vi "Image Analysis.vi"() -> ()   [LabVIEW 2010]
uses:
  <vilib>/Utility/miscctls.llb/LVMouseTypeDef.ctl
  <vilib>/Analysis/2dsp.llb/2D Real FFT.vi
  <vilib>/Analysis/2dsp.llb/2D Inverse Real FFT.vi
  <vilib>/picture/picture.llb/Draw True-Color Pixmap.vi
  <vilib>/Analysis/NI_AALPro.lvlib
  <vilib>/Analysis/NI_AALBase.lvlib
panel:
  in  "System Refresh Button":bool
  in  "Clear Image":bool
  in  "Find Atoms":bool
  in  "Save Marked Image":bool
  in  "index":i32
  in  "Pixel intensity":u8[][](array[numeric])
  out "Numeric 2":i32
  out "Numeric":i32
  in  "Tab Control 2":enum32{"Page 1", "Page 2"}(tab)
  in  "Local Max":bool
  in  "Pixel Radius":i32
  in  "Cutoff":dbl(slide)=0.9219858156028369 scale=0.0..1.0
  in  "STEM Image":path
  out "History Data":T1(array[cluster])
  in  "Tab Control":enum32{"Image", "FFT", "Analysis", "Advanced"}(tab)
  out "Working Image":picture
  in  "Zoom":dbl(slide)=0.9832134292565947 scale=0.0..20.0
  in  "Color":u32(colorbox)=16726826
  out "Angle (Degrees)":dbl
  out "Cos (Theta)":dbl
  in  "System Stop Button":bool
  out "Cropped Image":picture
  out "FFT":picture
  in  "Zoom 2":dbl(slide)=1.079136690647482 caption="Zoom" scale=0.0..10.0
  in  "Noise Factor":dbl(slide) scale=0.0..2.0
  in  "Xlength":i32(slide)=1024 scale=0.0..1024.0
  in  "YLength":i32(slide)=1024
  in  "X":i32
  in  "Y":i32
  in  "Mod":i32
  in  "Max X":dbl(slide) scale=0.0..1024.0
  in  "MAx Y":dbl
  out "RSD (%)":dbl format="%#_g%%"
  out "Std Dev":dbl
  out "Average Angle (Deg)":dbl
  out "Histogram Graph":T2(graph)
  out "Histogram Graph 2":T2(graph)
  out "Angles":T3(graph)
  in  "intervals":i32(slide)=10 scale=0.0..10.0
  out "RSD (%) 2":dbl format="%#_g%%"
  out "Std Dev 2":dbl
  out "Average Angle (Deg) 2":dbl
  in  "Slice Index":i32=24
  out "Atom Positions":T4(array[cluster])
  out "Last Last Mouse Pos":cluster{"Mouse X":i32, "Mouse Y":i32}
  out "Last Mouse Position":cluster{"Mouse X":i32, "Mouse Y":i32}={"Mouse X"=-1, "Mouse Y"=-1}
  out "CdTe Position Vector":dbl[](array[numeric])
  out "Mouse":T5={"Mouse Position"={"X"=21, "Y"=535}, "Mouse Modifiers"={"Button Down"=FALSE, "Shift Mod"=FALSE, "Menu Mod"=FALSE, "Option Mod"=FALSE}}
  out "Original Image":picture
  # "Drag and drop an Image here"
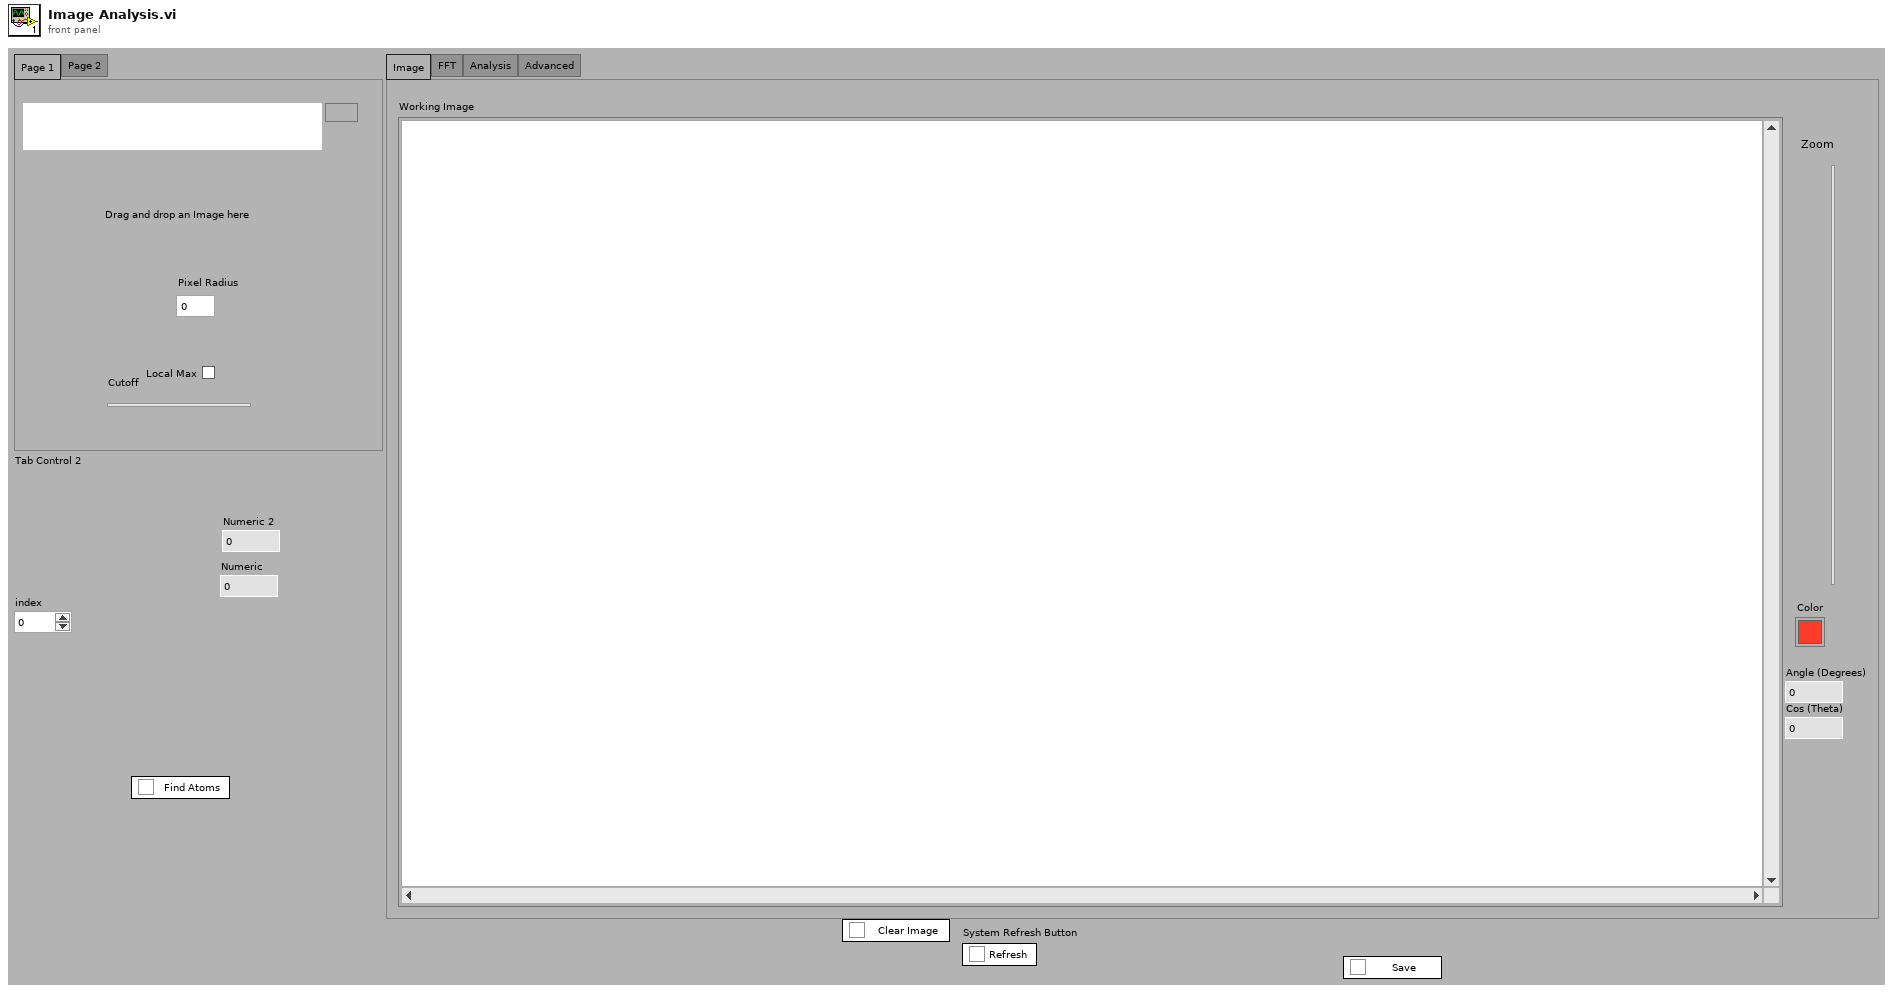
[diagram p1: front panel]
types:
  T1 = cluster{"Angle (Degrees)":dbl, "Cos (Theta)":dbl}[]
  T2 = cluster{"X Values":dbl[], "Histogram: h(x)":i32[]}
  T3 = cluster{"Angle (Degrees)":dbl, "Cos (Theta)":dbl}
  T4 = cluster{"Atom":string, "Pixel X":i32, "Pixel Y":i32}[]
  T5 = typedef "LVMouseTypeDef.ctl" = cluster{"Mouse Position":cluster{"X":i32, "Y":i32}, "Mouse Modifiers":cluster{"Button Down":bool, "Shift Mod":bool, "Menu Mod":bool, "Option Mod":bool}}
  T6 = cluster{"Width":u16, "Style":enum32{"Solid", "Dash", "Dot", "DashDot", "DashDotDot"}}
  T7 = typedef "imagedata.ctl" = cluster{"image type":i32, "image depth":i32, "image":u8[], "mask":u8[], "colors":u32[], "Rectangle":cluster{"left":i16, "top":i16, "right":i16, "bottom":i16}}
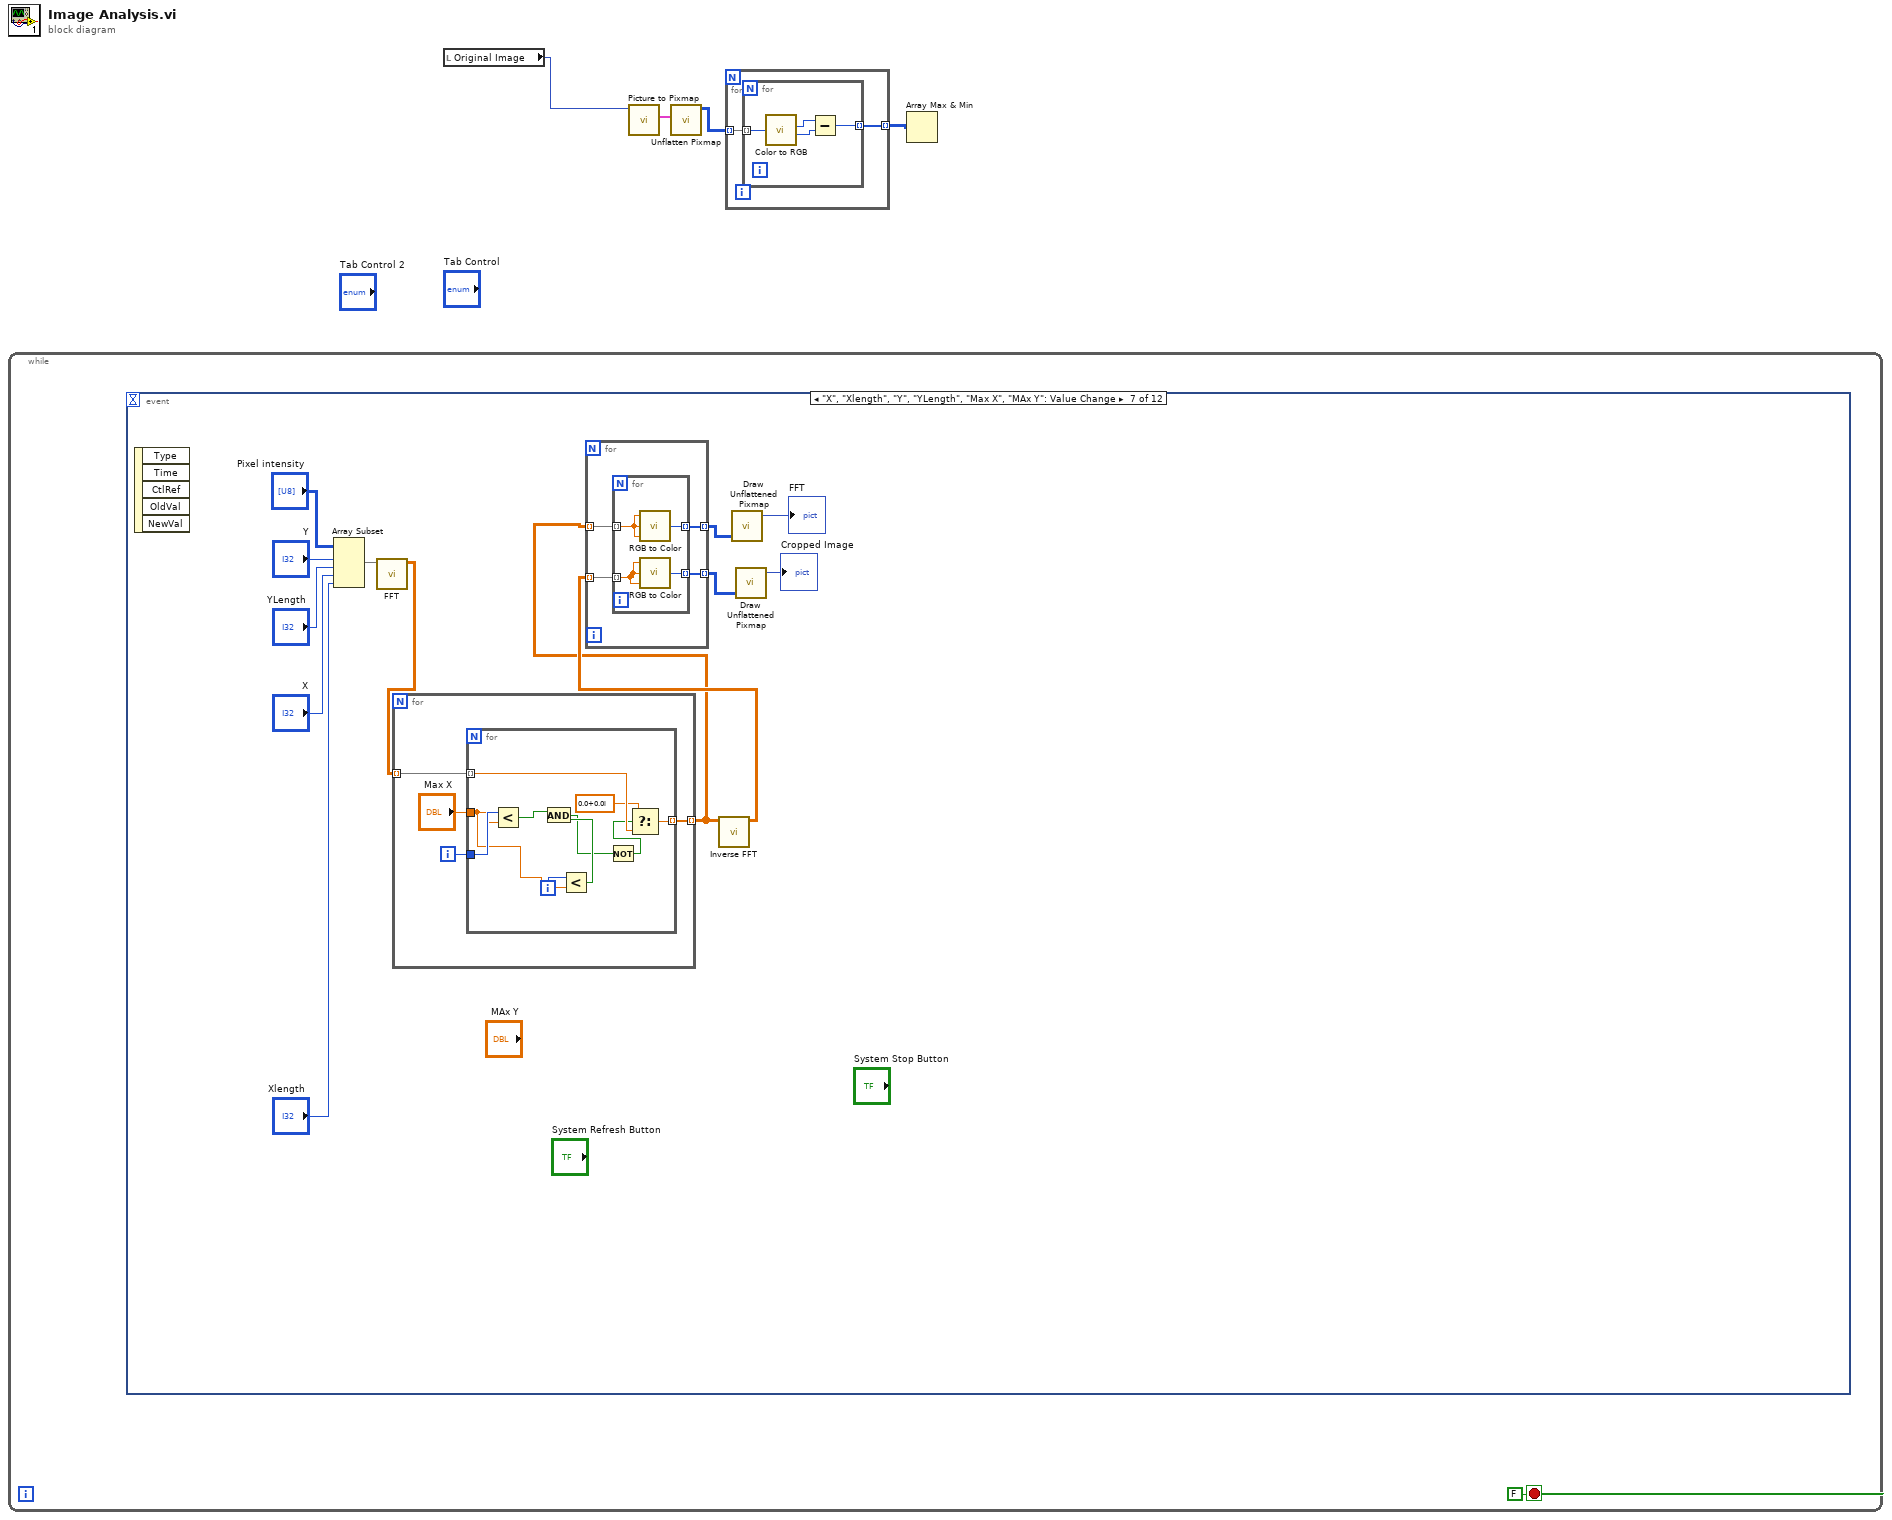
[diagram p0: block diagram]
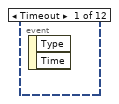
[diagram p2: hidden frame]
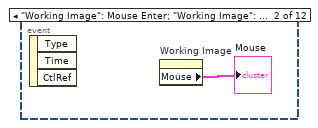
[diagram p3: hidden frame]
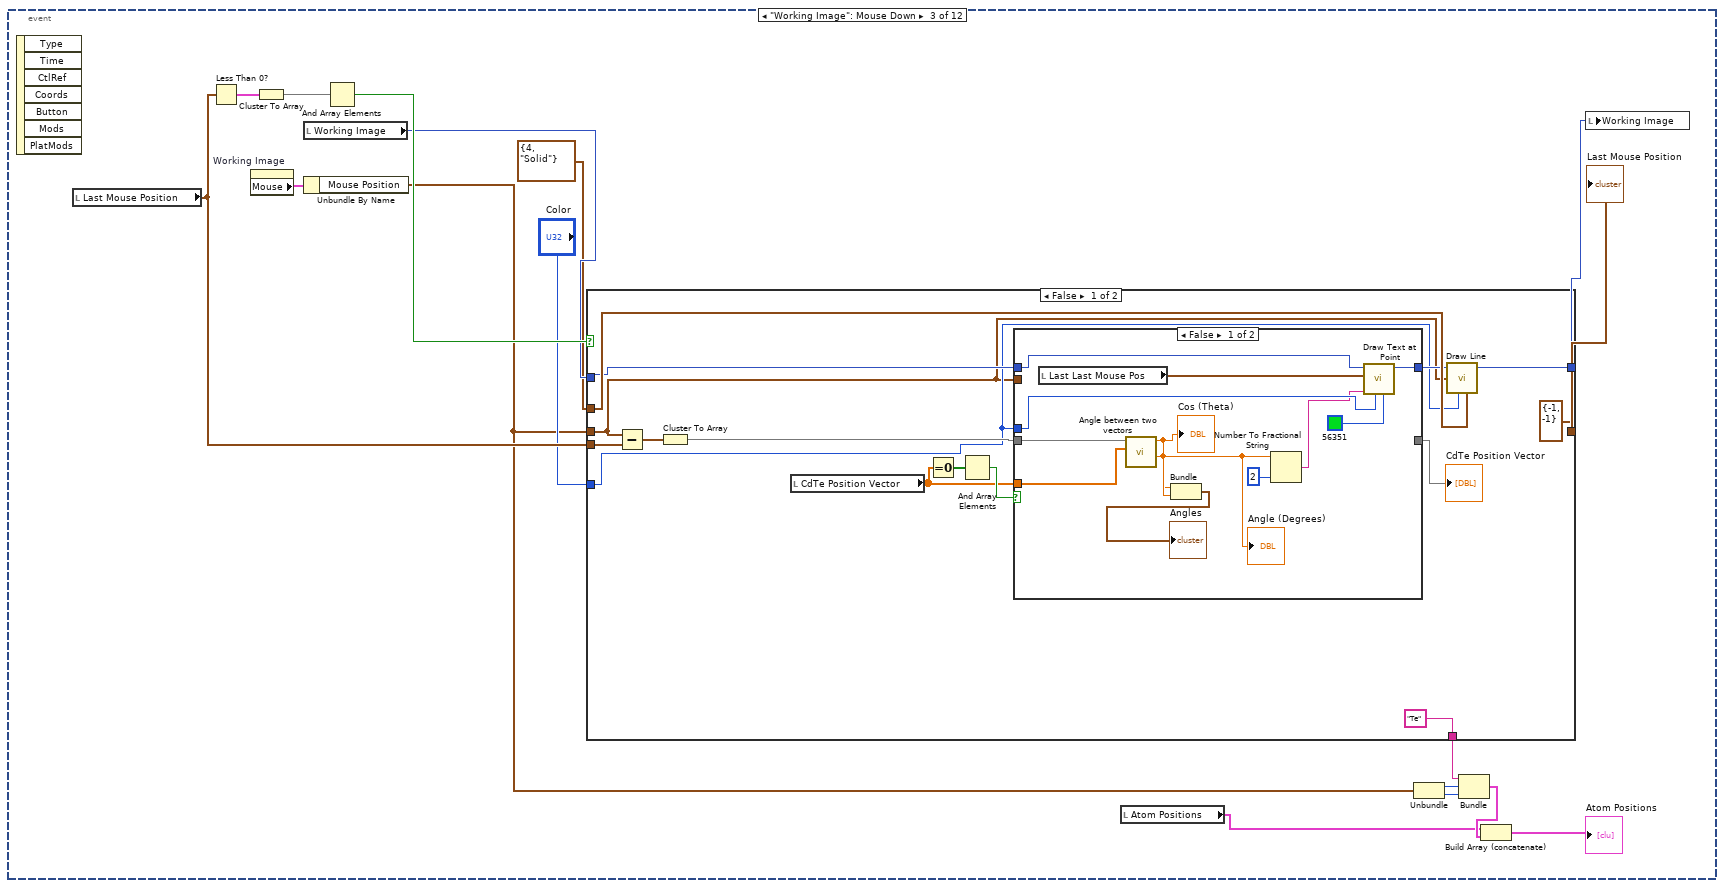
[diagram p4: hidden frame]
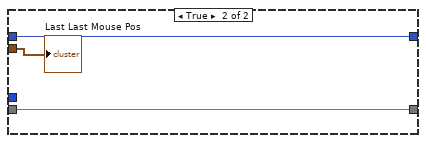
[diagram p5: hidden frame]
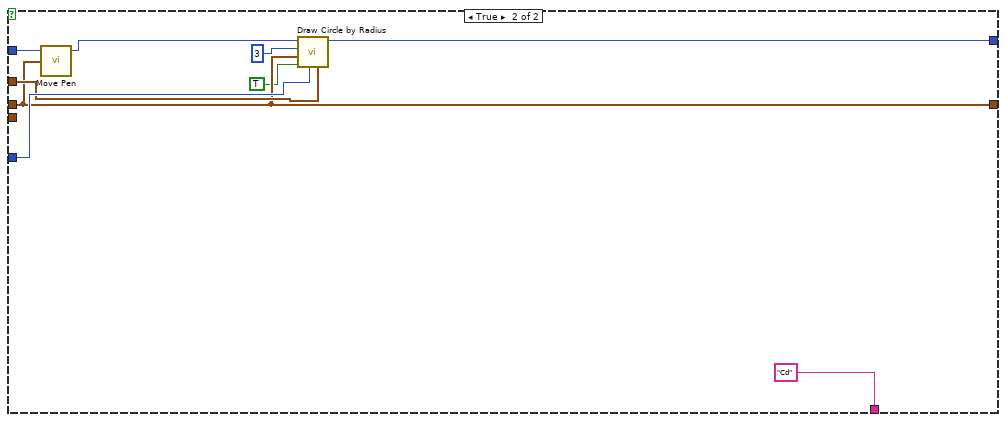
[diagram p6: hidden frame]
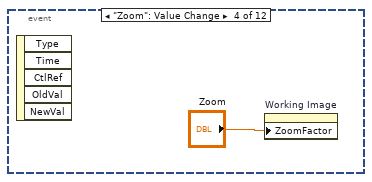
[diagram p7: hidden frame]
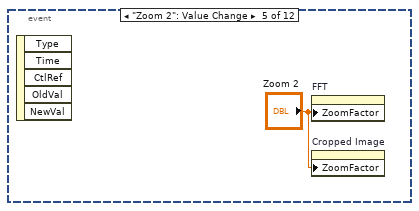
[diagram p8: hidden frame]
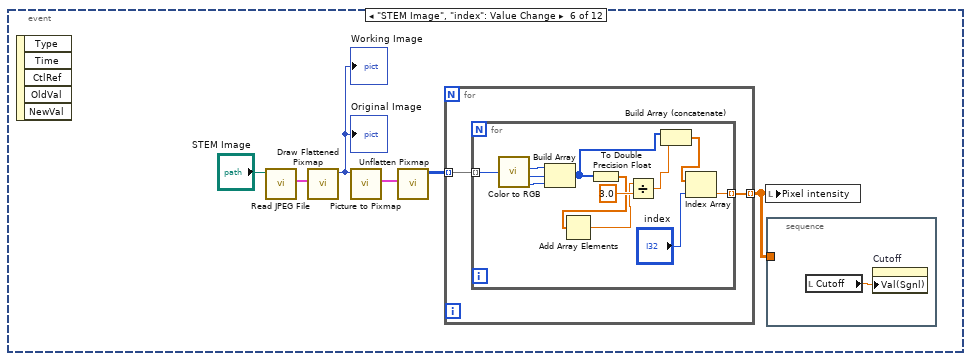
[diagram p9: hidden frame]
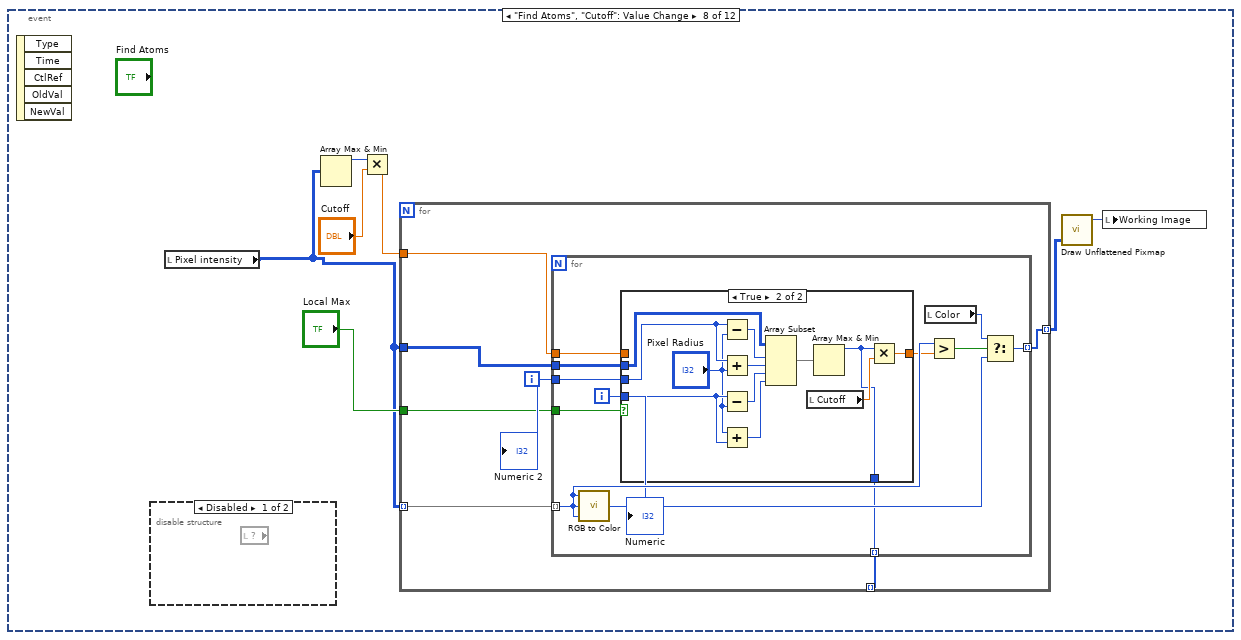
[diagram p10: hidden frame]
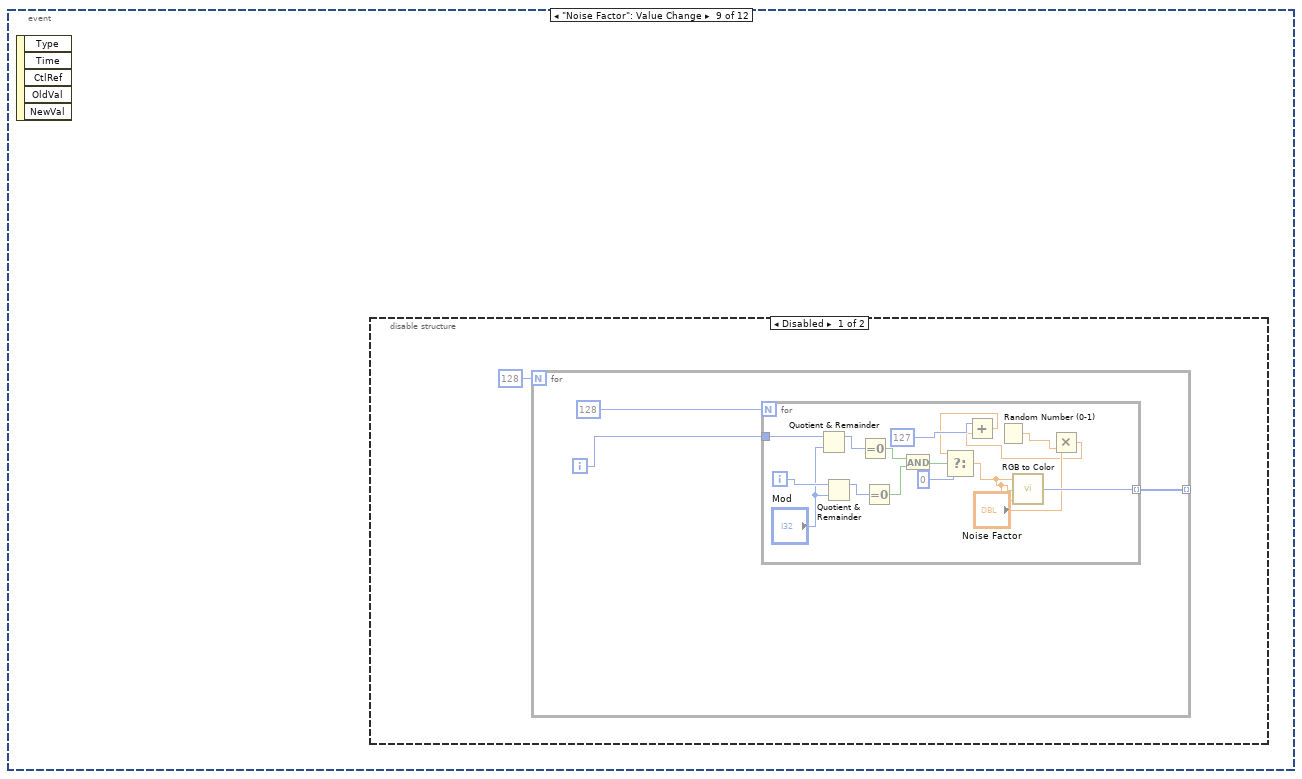
[diagram p13: hidden frame]
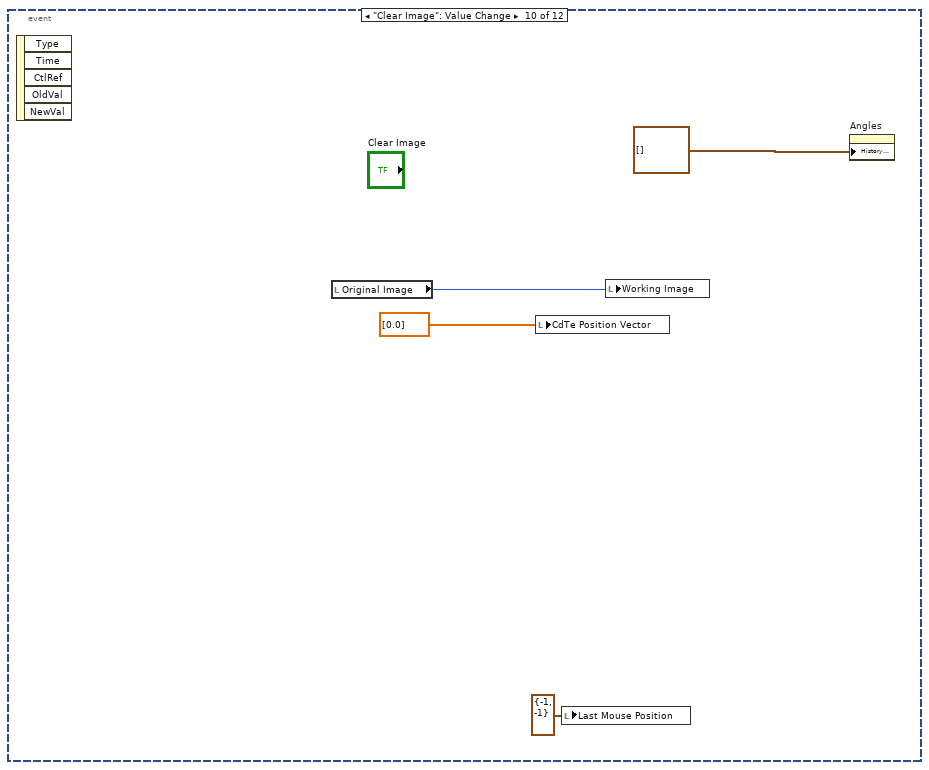
[diagram p15: hidden frame]
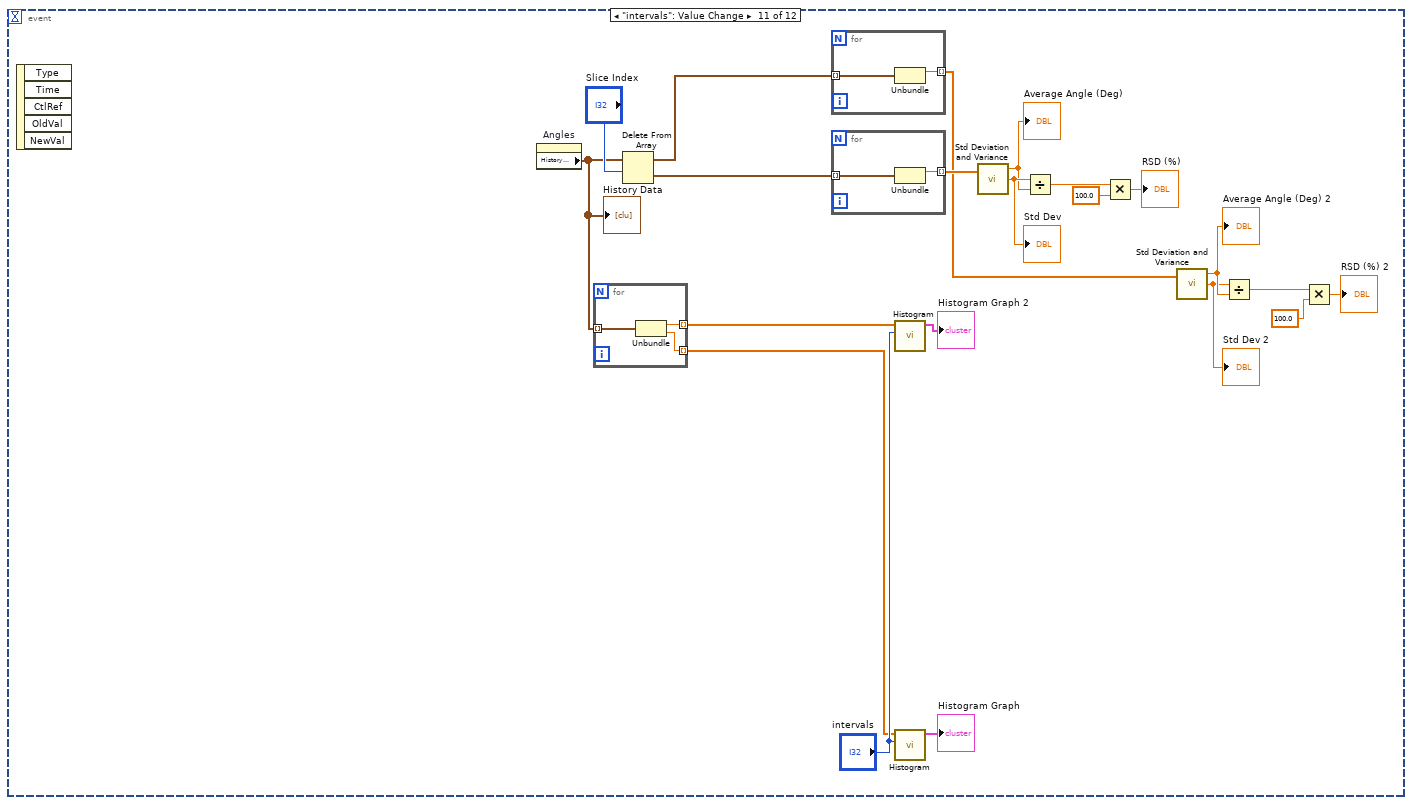
[diagram p16: hidden frame]
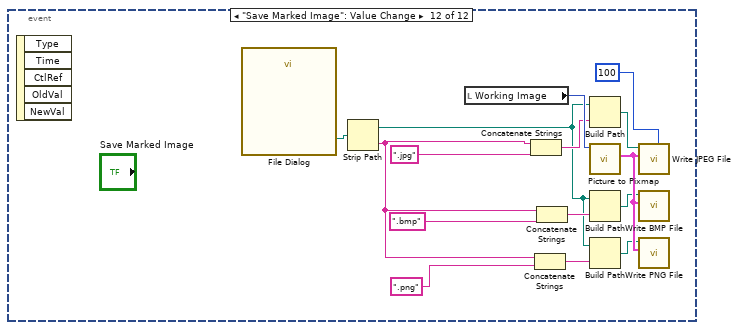
[diagram p17: hidden frame]
diagram:
  n1 = while {
    stop <- FALSE stop-if-true
    n2 = event shown="[6] \"X\", \"Xlength\", \"Y\", \"YLength\", \"Max X\", \"MAx Y\": Value Change" {
      selector: _ -> [_ _ _ _ _ _ _ _ _ _ _ _]
      dyn-events: _ -> [_ _ _ _ _ _ _ _ _ _ _ _]
      timeout: _ -> [_ _ _ _ _ _ _ _ _ _ _ _]
      event Timeout {
        n3 = event-data() -> ()  [unwired: 1 in, 2 out]
      }
      event "Working Image": Mouse Enter; "Working Image": Mouse Move {
        n4 = event-data() -> ()  [unwired: 1 in, 3 out]
        n5 = property on="Working Image" class="Pict"() -> ("Mouse"=→"Mouse":T5)  [unwired: 2 in, 2 out]
      }
      event "Working Image": Mouse Down {
        n6 = event-data() -> ()  [unwired: 1 in, 7 out]
        n7 = local read "Last Mouse Position"() -> (w20:cluster{"Mouse X":i32, "Mouse Y":i32})
        n8 = Less Than 0?(x=w20) -> (x < 0?=w23:cluster{"Mouse X":bool, "Mouse Y":bool})
        n9 = property on="Working Image" class="Pict"() -> ("Mouse"=w18:T5)  [unwired: 2 in, 2 out]
        n10 = Cluster To Array(cluster=w23) -> (array=w22:bool[])
        n11 = local read "Working Image"() -> (w17:picture)
        n12 = Unbundle By Name(w18) -> ("Mouse Position"=w12:cluster{"X":i32, "Y":i32})
        n13 = And Array Elements(Boolean array=w22) -> (logical AND=w21:bool)
        n14 = case shown="False" w21 {
          tunnel: w20 -> [w38 _]
          tunnel: [cluster{"X":i32, "Y":i32} {"X"=-1, "Y"=-1} ("Mouse Position") w57] -> w19
          tunnel: w12 -> [w26 w57]
          tunnel: w17 -> [w29 w59]
          tunnel: [w31 w62] -> w16
          tunnel: "Color" -> [w27 w61]
          tunnel: T6 {"Width"=4, "Style"=enum."Solid"} ("pen") -> [w30 w60]
          tunnel: ["Te" "Cd"] -> w13
          frame False {
            n15 = Subtract(x=w26, y=w38) -> (x-y=w35:cluster{i32, i32})
            n16 = Cluster To Array(cluster=w35) -> (array=w32:i32[])
            n17 = local read "CdTe Position Vector"() -> (w36:dbl[])
            n18 = Equal To 0?(x=w36) -> (x = 0?=w33:bool[])
            n19 = And Array Elements(Boolean array=w33) -> (logical AND=w37:bool)
            n20 = case shown="False" w37 {
              tunnel: w36 -> [w49 _]
              tunnel: w32 -> [w50 w53]
              tunnel: [_ w53] -> w34
              tunnel: w29 -> [w48 w52]
              tunnel: [w47 w52] -> w28
              tunnel: w27 -> [w46 _]
              tunnel: w26 -> [_ w51]
              frame False {
                n21 = local read "Last Last Mouse Pos"() -> (w42:cluster{"Mouse X":i32, "Mouse Y":i32})
                n22 = call "Angle between two vectors.vi"("Vector 2"=w49, "Vector 1"=w50) -> ("Angle (Degrees)"=w40:dbl, "Cos (Theta)"=w41:dbl)  [unwired: 7 in, 1 out]
                "Angle (Degrees)" <- w40
                "Cos (Theta)" <- w41
                n23 = Bundle("Angle (Degrees)"=w40, "Cos (Theta)"=w41) -> (→"Angles":T3)  [unwired: 1 in]
                n24 = Number To Fractional String(number=w40, precision (6)=i16 2) -> (F-format string=w43:string)  [unwired: 2 in]
                n25 = call <vilib>:"Draw Text at Point.vi"("BG color(transparent)"=u32 56351, "text color(black)"=w46, "text"=w43, "origin"=w42, "picture"=w48) -> ("new picture"=w47:picture)  [unwired: 5 in, 1 out]
              }
              frame True {
                "Last Last Mouse Pos" <- w51
              }
            }
            "CdTe Position Vector" <- w34
            n26 = call <vilib>:"Draw Line.vi"("picture"=w28, "end point"=w26, "color(black)"=w27, "pen"=w30) -> ("new picture"=w31:picture)  [unwired: 5 in]
          }
          frame True {
            n27 = call <vilib>:"Move Pen.vi"("new position"=w57, "picture"=w59) -> ("new picture"=w58:picture)  [unwired: 3 in]
            n28 = call <vilib>:"Draw Circle by Radius.vi"("pen"=w60, "color(black)"=w61, "fill?(F)"=TRUE, "pixel center"=w57, "radius"=i16 3, "picture"=w58) -> ("new picture"=w62:picture)  [unwired: 5 in]
          }
        }
        "Last Mouse Position" <- w19
        n29 = local read "Atom Positions"() -> (w8:T4)
        n30 = Unbundle(w12) -> ("X"=w11:i32, "Y"=w10:i32)
        n31 = Bundle(w13, "X"=w11, "Y"=w10) -> (w9:cluster{string, "X":i32, "Y":i32})  [unwired: 1 in]
        n32 = Build Array (concatenate)(w8, w9) -> (→"Atom Positions":cluster{"Atom":string, "X":i32, "Y":i32}[])
        n33 = local write "Working Image"(w16) -> ()
      }
      event "Zoom": Value Change {
        n34 = event-data() -> ()  [unwired: 1 in, 5 out]
        n35 = property on="Working Image" class="Pict"("ZoomFactor"="Zoom") -> ()  [unwired: 2 in, 2 out]
      }
      event "Zoom 2": Value Change {
        n36 = event-data() -> ()  [unwired: 1 in, 5 out]
        n37 = property on="FFT" class="Pict"("ZoomFactor"="Zoom 2") -> ()  [unwired: 2 in, 2 out]
        n38 = property on="Cropped Image" class="Pict"("ZoomFactor"="Zoom 2") -> ()  [unwired: 2 in, 2 out]
      }
      event "STEM Image", "index": Value Change {
        n39 = event-data() -> ()  [unwired: 1 in, 5 out]
        n40 = call <vilib>:"Read JPEG File.vi"("path to JPEG file"="STEM Image") -> ("image data"=w69:T7)  [unwired: 8 in, 2 out]
        n41 = call <vilib>:"Draw Flattened Pixmap.vi"("image data"=w69) -> ("new picture"=w65:picture)  [unwired: 8 in]
        "Working Image" <- w65
        "Original Image" <- w65
        n42 = call <vilib>:"Picture to Pixmap.vi"("picture"=w65) -> ("image data"=w68:T7)  [unwired: 9 in, 1 out]
        n43 = call <vilib>:"Unflatten Pixmap.vi"("image data"=w68) -> ("24-bit pixmap"=w67:u32[][])  [unwired: 4 in, 6 out]
        n44 = for {
          tunnel: w67 -> [w73] mode=indexing
          tunnel: [w72] -> w66 mode=indexing
          n45 = for {
            tunnel: w73 -> [w85] mode=indexing
            tunnel: [w84] -> w72 mode=indexing
            n46 = call <vilib>:"Color to RGB.vi"("Color"=w85) -> ("R"=w82:u8, "G"=w81:u8, "B"=w80:u8)  [unwired: 1 out]
            n47 = Build Array(w82, w81, w80) -> (w78:u8[])
            n48 = To Double Precision Float(number=w78) -> (double precision float=w76:dbl[])
            n49 = Add Array Elements(numeric array=w76) -> (sum=w75:dbl)
            n50 = Divide(x=w75, y=3.0) -> (x/y=w77:dbl)
            n51 = Build Array (concatenate)(w78, w77) -> (w74:dbl[])
            n52 = Index Array(array=w74, index="index") -> (element=w84:dbl)
          }
        }
        n53 = local write "Pixel intensity"(w66) -> ()
        n54 = stacked-sequence {
          tunnel: w66 -> [_]
          frame #0 {
            n55 = local read "Cutoff"() -> (w71:dbl)
            n56 = property on="Cutoff" class="Slide (strict)"("Val(Sgnl)"=w71) -> ()  [unwired: 2 in, 2 out]
          }
        }
      }
      event "X", "Xlength", "Y", "YLength", "Max X", "MAx Y": Value Change {
        n57 = event-data() -> ()  [unwired: 1 in, 5 out]
        n58 = Array Subset(array="Pixel intensity", index (row)="Y", length (row)="YLength", index (col)="X", length (col)="Xlength") -> (w98:u8[][])
        n59 = call-poly <vilib>:"FFT.vi"("X"=w98) -> ("FFT {X}"=w88:cdb[][])  [unwired: 9 in, 1 out]
        n60 = for {
          tunnel: w88 -> [w102] mode=indexing
          tunnel: [w99] -> w86 mode=indexing
          i -> [w100]
          n61 = for {
            tunnel: w102 -> [w107] mode=indexing
            tunnel: "Max X" -> [w103]
            tunnel: w100 -> [w110]
            tunnel: [w108] -> w99 mode=indexing
            i -> [w109]
            n62 = Less?(x=w110, y=w103) -> (x < y?=w112:bool)
            n63 = Less?(x=w109, y=w103) -> (x < y?=w111:bool)
            n64 = And(x=w112, y=w111) -> (x .and. y?=w105:bool)
            n65 = Not(x=w105) -> (.not. x?=w104:bool)
            n66 = Select(t=cdb 0.0+0.0i, s=w104, f=w107) -> (s? t:f=w108:cdb)
          }
        }
        n67 = call-poly <vilib>:"Inverse FFT.vi"("FFT {X}"=w86) -> ("X"=w87:dbl[][])  [unwired: 9 in, 1 out]
        n68 = for {
          tunnel: w86 -> [w116] mode=indexing
          tunnel: [w115] -> w90 mode=indexing
          tunnel: [w114] -> w89 mode=indexing
          tunnel: w87 -> [w113] mode=indexing
          n69 = for {
            tunnel: w116 -> [w120] mode=indexing
            tunnel: [w119] -> w115 mode=indexing
            tunnel: [w118] -> w114 mode=indexing
            tunnel: w113 -> [w117] mode=indexing
            n70 = call <vilib>:"RGB to Color.vi"("B"=w120, "G"=w120, "R"=w120) -> ("Color"=w119:u32)
            n71 = call <vilib>:"RGB to Color.vi"("B"=w117, "G"=w117, "R"=w117) -> ("Color"=w118:u32)
          }
        }
        n72 = call-poly <vilib>:"Draw Unflattened Pixmap.vi"("data (RGB format)"=w90) -> ("new picture"=→"FFT":picture)  [unwired: 8 in]
        n73 = call-poly <vilib>:"Draw Unflattened Pixmap.vi"("data (RGB format)"=w89) -> ("new picture"=→"Cropped Image":picture)  [unwired: 8 in]
      }
      event "Find Atoms", "Cutoff": Value Change {
        n74 = event-data() -> ()  [unwired: 1 in, 5 out]
        n75 = disable-structure shown="Disabled" {
          frame Disabled {
            n76 = local read item#-1() -> ()  [unwired: 1 out]
          }
          frame Enabled {
          }
        }
        n77 = local read "Pixel intensity"() -> (w121:u8[][])
        n78 = Array Max & Min(array=w121) -> (max value=w127:u8)  [unwired: 3 out]
        n79 = Multiply(x=w127, y="Cutoff") -> (x*y=w125:dbl)
        n80 = for {
          tunnel: w121 -> [w134] mode=indexing
          tunnel: w125 -> [w133]
          tunnel: [w132] -> w124 mode=indexing
          tunnel: w121 -> [w131]
          tunnel: "Local Max" -> [w129]
          tunnel: [w128] -> _ mode=indexing
          i -> [w130]
          n81 = for {
            tunnel: w134 -> [w143] mode=indexing
            tunnel: w133 -> [w137]
            tunnel: [w145] -> w132 mode=indexing
            tunnel: w131 -> [w141]
            tunnel: w130 -> [w139]
            tunnel: w129 -> [w136]
            tunnel: [w135] -> w128 mode=indexing
            i -> [w140]
            n82 = call <vilib>:"RGB to Color.vi"("B"=w143, "G"=w143, "R"=w143) -> ("Color"=w144:u32)
            n83 = case shown="True" w136 {
              tunnel: w141 -> [_ w159]
              tunnel: w140 -> [_ w158]
              tunnel: w139 -> [_ w154]
              tunnel: [w147 w149] -> w138
              tunnel: w137 -> [w147 _]
              tunnel: [_ w148] -> w135
              frame False {
              }
              frame True {
                n84 = Subtract(x=w154, y="Pixel Radius") -> (x-y=w156:i32)
                n85 = Add(x=w154, y="Pixel Radius") -> (x+y=w152:i32)
                n86 = Subtract(x=w158, y="Pixel Radius") -> (x-y=w157:i32)
                n87 = Add(x="Pixel Radius", y=w158) -> (x+y=w155:i32)
                n88 = Array Subset(array=w159, index (row)=w156, length (row)=w152, index (col)=w157, length (col)=w155) -> (w151:u8[][])
                n89 = local read "Cutoff"() -> (w150:dbl)
                n90 = Array Max & Min(array=w151) -> (max value=w148:u8)  [unwired: 3 out]
                n91 = Multiply(x=w148, y=w150) -> (x*y=w149:dbl)
              }
            }
            n92 = local read "Color"() -> (w142:u32)
            n93 = Greater?(x=w143, y=w138) -> (0:w146:bool)
            n94 = Select(t=w142, s=w146, f=w144) -> (s? t:f=w145:u32)
            "Numeric" <- w140
          }
          "Numeric 2" <- w130
        }
        n95 = call-poly <vilib>:"Draw Unflattened Pixmap.vi"("data (RGB format)"=w124) -> ("new picture"=w123:picture)  [unwired: 8 in]
        n96 = local write "Working Image"(w123) -> ()
      }
      event "Noise Factor": Value Change {
        n97 = event-data() -> ()  [unwired: 1 in, 5 out]
        n98 = disable-structure shown="Disabled" {
          frame Disabled {
            n99 = for {
              N: 128 -> [_]
              tunnel: [w161] -> _ mode=indexing
              i -> [w162]
              n100 = for {
                N: 128 -> [_]
                tunnel: w162 -> [w179]
                tunnel: [w169] -> w161 mode=indexing
                i -> [w178]
                n101 = Quotient & Remainder(x=w179, y="Mod") -> (x-y*floor(x/y)=w176:i32)  [unwired: 1 out]
                n102 = Quotient & Remainder(x=w178, y="Mod") -> (x-y*floor(x/y)=w175:i32)  [unwired: 1 out]
                n103 = Equal To 0?(x=w176) -> (x = 0?=w174:bool)
                n104 = Equal To 0?(x=w175) -> (x = 0?=w173:bool)
                n105 = And(x=w174, y=w173) -> (x .and. y?=w172:bool)
                n106 = Random Number (0-1)() -> (number: 0 to 1=w166:dbl)
                n107 = Multiply(x="Noise Factor", y=w166) -> (x*y=w164:dbl)
                n108 = Add(x=u8 127 ("R"), y=w164) -> (x+y=w167:dbl)
                n109 = Select(t=w167, s=w172, f=u8 0) -> (s? t:f=w170:dbl)
                n110 = call <vilib>:"RGB to Color.vi"("B"=w170, "G"=w170, "R"=w170) -> ("Color"=w169:u32)
              }
            }
          }
          frame Enabled {
          }
        }
      }
      event "Clear Image": Value Change {
        n111 = event-data() -> ()  [unwired: 1 in, 5 out]
        n112 = local read "Original Image"() -> (w183:picture)
        n113 = local write "CdTe Position Vector"(dbl[] [0.0] ("CdTe Position Vector")) -> ()
        n114 = local write "Last Mouse Position"(cluster{"Mouse X":i32, "Mouse Y":i32} {"Mouse X"=-1, "Mouse Y"=-1} ("Last Mouse Position")) -> ()
        n115 = local write "Working Image"(w183) -> ()
        n116 = property on="Angles" class="WFChart (strict)"("History Data"=T1 []) -> ()  [unwired: 2 in, 2 out]
      }
      event "intervals": Value Change {
        n117 = event-data() -> ()  [unwired: 1 in, 5 out]
        n118 = property on="Angles" class="WFChart (strict)"() -> ("History Data"=w192:T1)  [unwired: 2 in, 2 out]
        "History Data" <- w192
        n119 = for {
          tunnel: w192 -> [w207] mode=indexing
          tunnel: [w206] -> w191 mode=indexing
          tunnel: [w205] -> w190 mode=indexing
          n120 = Unbundle(w207) -> ("Angle (Degrees)"=w206:dbl, "Cos (Theta)"=w205:dbl)
        }
        n121 = Delete From Array(array=w192, length="Slice Index") -> (deleted portion=w194:T1, array with subset deleted=w193:T1)  [unwired: 1 in]
        n122 = for {
          tunnel: w193 -> [w209] mode=indexing
          tunnel: [w208] -> w184 mode=indexing
          n123 = Unbundle(w209) -> ("Angle (Degrees)"=w208:dbl)  [unwired: 1 out]
        }
        n124 = for {
          tunnel: w194 -> [w211] mode=indexing
          tunnel: [w210] -> w201 mode=indexing
          n125 = Unbundle(w211) -> ("Angle (Degrees)"=w210:dbl)  [unwired: 1 out]
        }
        n126 = call <vilib>:"Histogram.vi"("intervals"="intervals", "X"=w191) -> ("Histogram Graph"=→"Histogram Graph 2":T2)  [unwired: 6 in, 3 out]
        n127 = call <vilib>:"Histogram.vi"("intervals"="intervals", "X"=w190) -> ("Histogram Graph"=→"Histogram Graph":T2)  [unwired: 6 in, 3 out]
        n128 = call <vilib>:"Std Deviation and Variance.vi"("X"=w201) -> ("mean"=w199:dbl, "standard deviation"=w200:dbl)  [unwired: 1 in, 1 out]
        "Average Angle (Deg)" <- w199
        "Std Dev" <- w200
        n129 = Divide(x=w200, y=w199) -> (x/y=w198:dbl)
        n130 = Multiply(x=w198, y=100.0) -> (x*y=→"RSD (%)":dbl)
        n131 = call <vilib>:"Std Deviation and Variance.vi"("X"=w184) -> ("mean"=w186:dbl, "standard deviation"=w185:dbl)  [unwired: 1 in, 1 out]
        "Average Angle (Deg) 2" <- w186
        "Std Dev 2" <- w185
        n132 = Divide(x=w185, y=w186) -> (x/y=w187:dbl)
        n133 = Multiply(x=w187, y=100.0) -> (x*y=→"RSD (%) 2":dbl)
      }
      event "Save Marked Image": Value Change {
        n134 = event-data() -> ()  [unwired: 1 in, 5 out]
        n135 = call "File Dialog"() -> ("selected path"=w223:path)  [unwired: 12 in, 3 out]
        n136 = Strip Path(path=w223) -> (stripped path=w212:path, name=w216:string)
        n137 = local read "Working Image"() -> (w226:picture)
        n138 = Concatenate Strings(w216, ".jpg" ("string")) -> (w222:string)
        n139 = Concatenate Strings(w216, ".png" ("string")) -> (w220:string)
        n140 = Concatenate Strings(w216, ".bmp" ("string")) -> (w221:string)
        n141 = Build Path(base path=w212, name or relative path=w222) -> (appended path=w215:path)
        n142 = call <vilib>:"Picture to Pixmap.vi"("picture"=w226) -> ("image data"=w224:T7)  [unwired: 9 in, 1 out]
        n143 = Build Path(base path=w212, name or relative path=w221) -> (appended path=w214:path)
        n144 = Build Path(base path=w212, name or relative path=w220) -> (appended path=w213:path)
        n145 = call <vilib>:"Write JPEG File.vi"("quality (80)"=100, "image data"=w224, "path to JPEG file"=w215) -> ()  [unwired: 7 in, 2 out]
        n146 = call <vilib>:"Write BMP File.vi"("image data"=w224, "path to BMP file"=w214) -> ()  [unwired: 8 in, 2 out]
        n147 = call <vilib>:"Write PNG File.vi"("image data"=w224, "path to PNG file"=w213) -> ()  [unwired: 8 in, 2 out]
      }
    }
  }
  n148 = local read "Original Image"() -> (w1:picture)
  n149 = call <vilib>:"Picture to Pixmap.vi"("picture"=w1) -> ("image data"=w4:T7)  [unwired: 9 in, 1 out]
  n150 = call <vilib>:"Unflatten Pixmap.vi"("image data"=w4) -> ("24-bit pixmap"=w3:u32[][])  [unwired: 4 in, 6 out]
  n151 = for {
    tunnel: w3 -> [w228] mode=indexing
    tunnel: [w227] -> w2 mode=indexing
    n152 = for {
      tunnel: w228 -> [w232] mode=indexing
      tunnel: [w229] -> w227 mode=indexing
      n153 = call <vilib>:"Color to RGB.vi"("Color"=w232) -> ("R"=w231:u8, "G"=w230:u8)  [unwired: 2 out]
      n154 = Subtract(x=w231, y=w230) -> (x-y=w229:u8)
    }
  }
  n155 = Array Max & Min(array=w2) -> ()  [unwired: 4 out]
